vi "phase to compensation (host).vi"(10 "phases":T1) -> (2 "for comp":T2={"channel 1 "={"Real"=1.0, "Imag"=0.0}, "channel  2"={"Real"=1.0, "Imag"=0.0}, "channel  3"={"Real"=1.0, "Imag"=0.0}, "channel  4"={"Real"=1.0, "Imag"=0.0}})   [LabVIEW 2020]
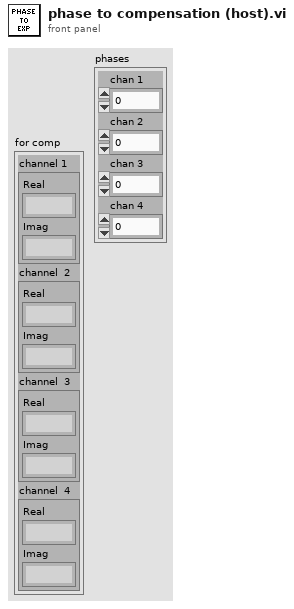
[diagram p1: front panel]
types:
  T1 = cluster{"chan 1":dbl, "chan 2":dbl, "chan 3":dbl, "chan 4":dbl}
  T2 = cluster{"channel 1 ":cluster{"Real":fxp<+/-,16,3>, "Imag":fxp<+/-,16,3>}, "channel  2":cluster{"Real":fxp<+/-,16,3>, "Imag":fxp<+/-,16,3>}, "channel  3":cluster{"Real":fxp<+/-,16,3>, "Imag":fxp<+/-,16,3>}, "channel  4":cluster{"Real":fxp<+/-,16,3>, "Imag":fxp<+/-,16,3>}}
  T3 = cluster{"Real":fxp<+/-,16,3>, "Imag":fxp<+/-,16,3>}
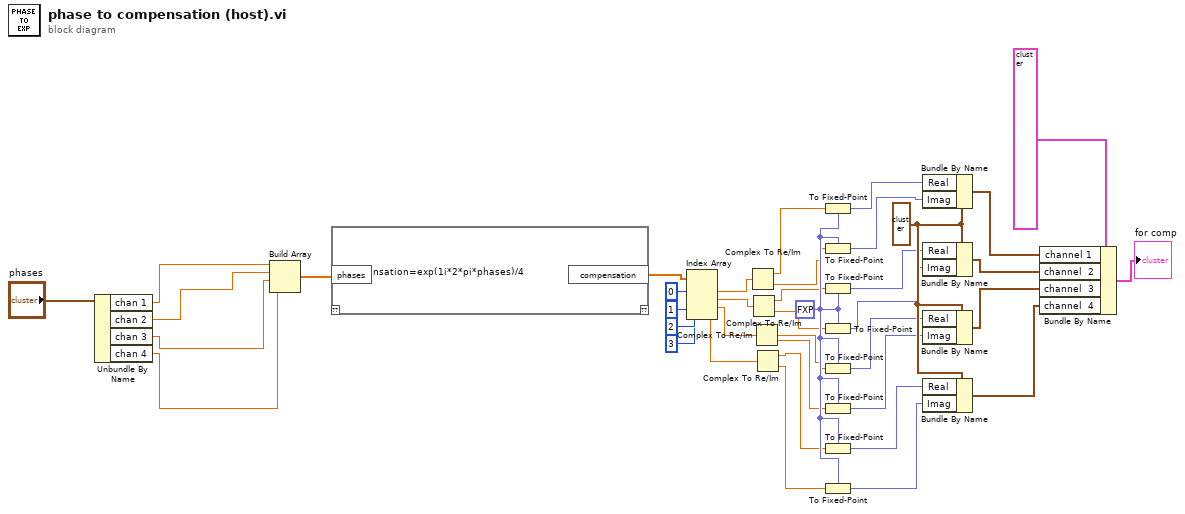
[diagram p0: block diagram]
diagram:
  w26 = fxp<+/-,16,3> 0.0 ("Real")
  w21 = T3 {"Real"=1.0, "Imag"=0.0} ("channel  3")
  n1 = Unbundle By Name("phases") -> ("chan 1"=w4:dbl, "chan 2"=w3:dbl, "chan 3"=w2:dbl, "chan 4"=w1:dbl)
  n2 = Build Array(w4, w3, w2, w1) -> (w39:dbl[])
  n3 = script code="compensation=exp(1i*2*pi*phases)/4"("phases"=w39) -> ("compensation"=w38:cdb[])  [unwired: 1 in, 1 out]
  n4 = Index Array(array=w38, index #1=0 ("index"), index #2=1 ("index"), index #3=2 ("index"), index #4=3 ("index")) -> (element #1=w33:cdb, element #2=w32:cdb, element #3=w31:cdb, element #4=w30:cdb)
  n5 = Complex To Re/Im(x + iy=w33) -> (x=w29:dbl, y=w20:dbl)
  n6 = Complex To Re/Im(x + iy=w32) -> (x=w19:dbl, y=w18:dbl)
  n7 = Complex To Re/Im(x + iy=w31) -> (x=w17:dbl, y=w16:dbl)
  n8 = Complex To Re/Im(x + iy=w30) -> (x=w15:dbl, y=w14:dbl)
  n9 = To Fixed-Point(fixed-point type=w26, number=w29) -> (fixed-point=w13:fxp<+/-,16,3>)
  n10 = To Fixed-Point(fixed-point type=w26, number=w20) -> (fixed-point=w12:fxp<+/-,16,3>)
  n11 = To Fixed-Point(fixed-point type=w26, number=w19) -> (fixed-point=w11:fxp<+/-,16,3>)
  n12 = To Fixed-Point(fixed-point type=w26, number=w18) -> (fixed-point=w10:fxp<+/-,16,3>)
  n13 = To Fixed-Point(fixed-point type=w26, number=w17) -> (fixed-point=w9:fxp<+/-,16,3>)
  n14 = To Fixed-Point(fixed-point type=w26, number=w16) -> (fixed-point=w8:fxp<+/-,16,3>)
  n15 = To Fixed-Point(fixed-point type=w26, number=w15) -> (fixed-point=w7:fxp<+/-,16,3>)
  n16 = To Fixed-Point(fixed-point type=w26, number=w14) -> (fixed-point=w6:fxp<+/-,16,3>)
  n17 = Bundle By Name(cluster=w21, "Real"=w13, "Imag"=w12) -> (w25:T3)
  n18 = Bundle By Name(cluster=w21, "Real"=w11, "Imag"=w10) -> (w24:T3)
  n19 = Bundle By Name(cluster=w21, "Real"=w9, "Imag"=w8) -> (w22:T3)
  n20 = Bundle By Name(cluster=w21, "Real"=w7, "Imag"=w6) -> (w23:T3)
  n21 = Bundle By Name(cluster=T2 {"channel 1 "={"Real"=1.0, "Imag"=0.0}, "channel  2"={"Real"=1.0, "Imag"=0.0}, "channel  3"={"Real"=1.0, "Imag"=0.0}, "channel  4"={"Real"=1.0, "Imag"=0.0}} ("compensation"), "channel 1"=w25, "channel  2"=w24, "channel  3"=w22, "channel  4"=w23) -> (→"for comp":T2)
